vi "LabViewAnirban.vi"() -> ()   [LabVIEW 2019]
uses:
  <vilib>/addons/control/pid/pid.llb/PID (DBL).vi
  <vilib>/addons/control/pid/NI_PID_pid.lvlib
panel:
  out "elapsed time (ms)":dbl
  out "Waveform Chart":dynamicdata(graph)
  in  "stop":bool
  in  "PID gains":T1={"proportional gain (Kc)"=1.0, "integral time (Ti, min)"=0.01, "derivative time (Td, min)"=0.0} {"derivative time (Td, min)" format="%.7f"; "integral time (Ti, min)" format="%.7f"; "proportional gain (Kc)" format="%.3f"}
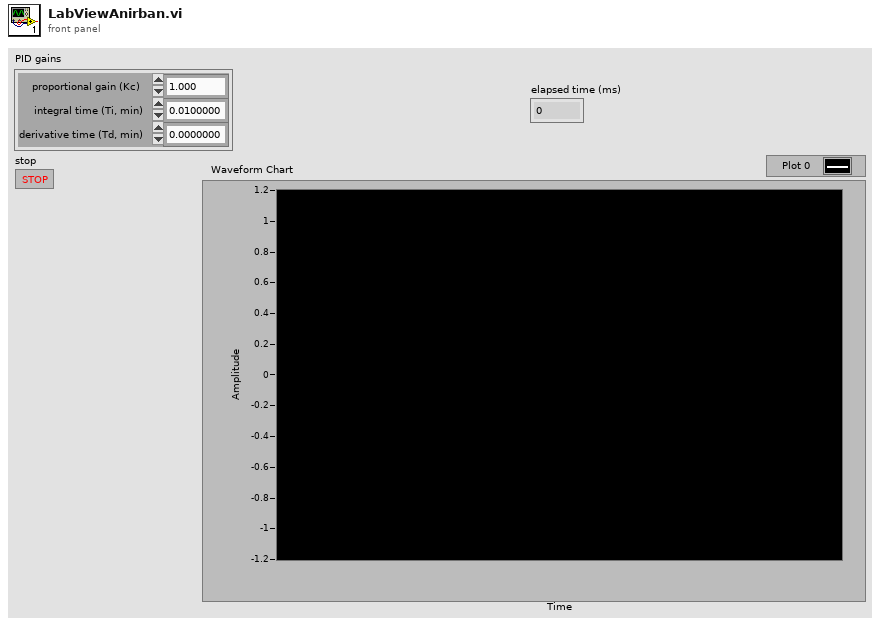
[diagram p1: front panel]
types:
  T1 = cluster{"proportional gain (Kc)":dbl, "integral time (Ti, min)":dbl, "derivative time (Td, min)":dbl}
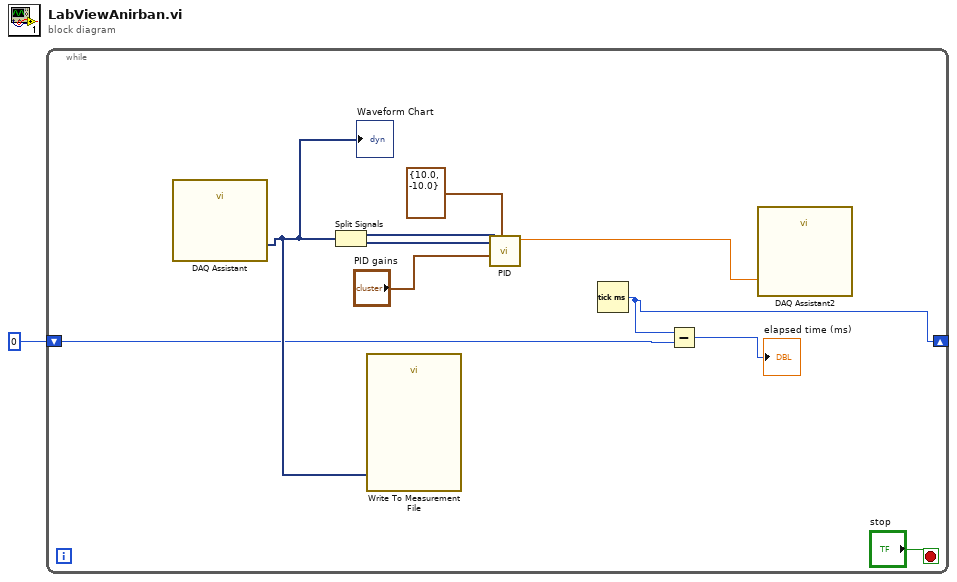
[diagram p0: block diagram]
diagram:
  n1 = while {
    shift-right: [w3] -> _
    shift-left: 0 -> [w2]
    stop <- "stop" stop-if-true
    n2 = call "DAQ Assistant"() -> ("data"=w5:dynamicdata)  [unwired: 17 in, 2 out]
    "Waveform Chart" <- w5
    n3 = Split Signals(w5) -> (w11:dynamicdata, w10:dynamicdata)  [unwired: 2 in]
    n4 = call "Write To Measurement File"("Signals"=w5) -> ()  [unwired: 16 in, 3 out]
    n5 = call-poly <vilib>:"PID.vi"("output range"=cluster{"output high":dbl, "output low":dbl} {"output high"=10.0, "output low"=-10.0}, "PID gains"="PID gains", "process variable"=w10, "setpoint"=w11) -> ("output"=w7:dbl)  [unwired: 6 in, 1 out]
    n6 = Tick Count (ms)() -> (millisecond timer value=w3:u32)
    n7 = Subtract(x=w3, y=w2) -> (x-y=→"elapsed time (ms)":u32)
    n8 = call "DAQ Assistant2"("data"=w7) -> ()  [unwired: 17 in, 2 out]
  }
